vi "pullPatchByArc_v02.vi"(0 "manp in":T2={"Actuator COM"="COM6", "Actuator type"=enum."Scientifica"}, 1 "reset motion":T1=enum."slow_dualPatch", 5 "Current Position":i32[](array[numeric]), 7 "Steps":i32, 9 "Final Distance (steps)":i32, 11 "error in":errorcluster) -> (4 "manip out":T2={"Actuator COM"="COM14", "Actuator type"=enum."Scientifica"}, 15 "error out":errorcluster)   [LabVIEW 2019]
uses:
  pipette cleaning/pressure box/cleaning_soft/controls/actuator_cluster.ctl
  pipette cleaning/pressure box/cleaning_soft/controls/actuator_type.ctl
  controls/scope_motion.ctl
panel:
  out "positionSequence":i32[][](array[numeric])
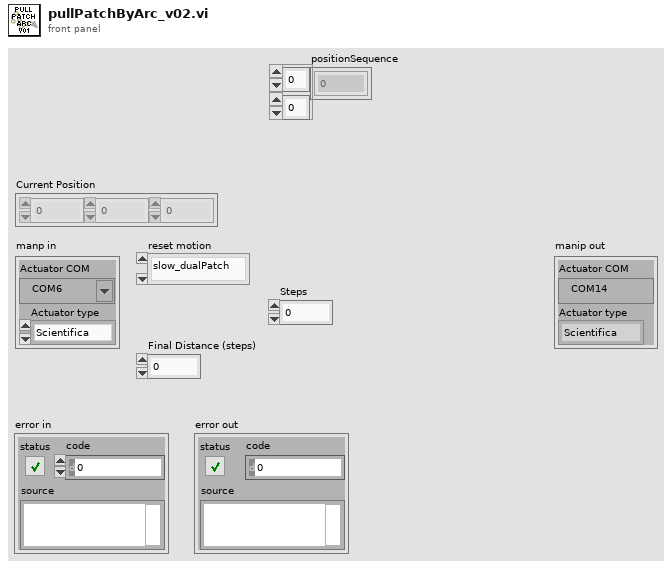
[diagram p1: front panel]
types:
  T1 = typedef "scope_motion.ctl" = enum16{"superSlow", "fast", "slow", "find slice speed", "slow_dualPatch"}
  T2 = typedef "actuator_cluster.ctl" = cluster{"Actuator COM":refnum<visa-resource-name>, "Actuator type":T3}
  T3 = typedef "actuator_type.ctl" = enum16{"Scientifica", "Sutter", "Demo", "Off"}
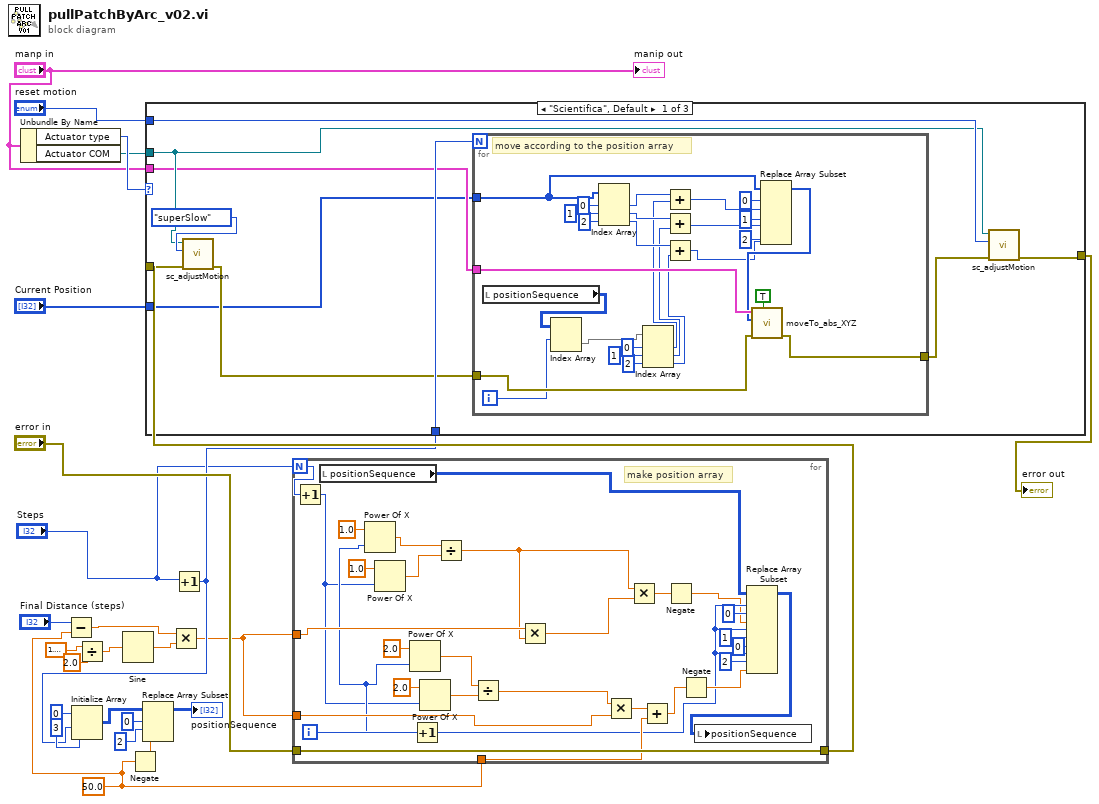
[diagram p0: block diagram]
diagram:
  w3 = 50.0 ("new element/subarray")
  n1 = Unbundle By Name("manp in") -> ("Actuator type"=w25:T3, "Actuator COM"=w24:refnum<visa-resource-name>)
  n2 = Subtract(x="Final Distance (steps)", y=w3) -> (x-y=w2:dbl)
  n3 = Divide(x=1.5707963267948966, y=2.0) -> (x/y=w12:dbl)
  n4 = Sine(x=w12) -> (sin(x)=w14:dbl)
  n5 = Negate(x=w3) -> (-x=w6:dbl)
  n6 = Multiply(x=w2, y=w14) -> (x*y=w8:dbl)
  n7 = Increment(x="Steps") -> (x+1=w9:i32)
  n8 = Initialize Array(0 ("element"), w9, 3 ("dimension size")) -> (w19:i32[][])
  n9 = Replace Array Subset(array=w19, new element=w6, index (row)=0 ("index"), index (col)=2 ("disabled index (col)")) -> (→"positionSequence":i32[][])
  n10 = for {
    N: "Steps" -> [w44]
    tunnel: w8 -> [w52]
    tunnel: "error in" -> [w50]
    tunnel: [w50] -> w10
    tunnel: w8 -> [w41]
    tunnel: w3 -> [w47]
    i -> [w43]
    # "make position array"
    n11 = Increment(x=w44) -> (x+1=w29:i32)
    n12 = local read "positionSequence"() -> (w49:i32[][])
    n13 = Power Of X(1:w29, 2:1.0 ("y")) -> (0:w34:dbl)
    n14 = Increment(x=w43) -> (x+1=w31:i32)
    n15 = Power Of X(1:w31, 2:1.0 ("y")) -> (0:w36:dbl)
    n16 = Power Of X(1:w31, 2:2.0 ("y")) -> (0:w30:dbl)
    n17 = Power Of X(1:w29, 2:2.0 ("y")) -> (0:w28:dbl)
    n18 = Divide(x=w36, y=w34) -> (x/y=w40:dbl)
    n19 = Divide(x=w30, y=w28) -> (x/y=w53:dbl)
    n20 = Multiply(x=w41, y=w40) -> (x*y=w39:dbl)
    n21 = Multiply(x=w53, y=w52) -> (x*y=w42:dbl)
    n22 = Multiply(x=w40, y=w39) -> (x*y=w48:dbl)
    n23 = Add(x=w42, y=w47) -> (x+y=w45:dbl)
    n24 = Negate(x=w48) -> (-x=w26:dbl)
    n25 = Negate(x=w45) -> (-x=w38:dbl)
    n26 = Replace Array Subset(array=w49, new element #1=w26, index (row) #1=w31, index (col) #1=0 ("index (row)"), new element #2=0 ("new element/subarray"), index (row) #2=w31, index (col) #2=1 ("disabled index (col)"), new element #3=w38, index (row) #3=w31, index (col) #3=2 ("disabled index (col)")) -> (w51:i32[][])
    n27 = local write "positionSequence"(w51) -> ()
  }
  n28 = case shown="\"Scientifica\", Default" w25 {
    tunnel: w24 -> [w61 _ _]
    tunnel: w10 -> [w65 w93 w94]
    tunnel: [w62 w93 w94] -> w22
    tunnel: "reset motion" -> [w64 _ _]
    tunnel: w9 -> [w60 _ _]
    tunnel: "Current Position" -> [w56 _ _]
    tunnel: "manp in" -> [w59 _ _]
    frame "Scientifica", Default {
      n29 = call "sc_adjustMotion.vi"("error in (no error)"=w65, "motion"=scope_motion."superSlow", "VISA handle"=w61) -> ("error out"=w58:errorcluster)  [unwired: 7 in, 1 out]
      n30 = for {
        N: w60 -> [_]
        tunnel: w59 -> [w92]
        tunnel: w58 -> [w90]
        tunnel: [w89] -> w57
        tunnel: w56 -> [w77]
        i -> [w79]
        # "move according to the position array"
        n31 = local read "positionSequence"() -> (w66:i32[][])
        n32 = Index Array(array=w66, index (row)=w79) -> (element=w73:i32[])  [unwired: 1 in]
        n33 = Index Array(array=w77, index #1=0 ("index"), index #2=1 ("index"), index #3=2 ("index")) -> (element #1=w82:i32, element #2=w81:i32, element #3=w80:i32)
        n34 = Index Array(array=w73, index #1=0 ("index"), index #2=1 ("index"), index #3=2 ("index")) -> (element #1=w70:i32, element #2=w72:i32, element #3=w71:i32)
        n35 = Add(x=w82, y=w70) -> (x+y=w67:i32)
        n36 = Add(x=w81, y=w72) -> (x+y=w68:i32)
        n37 = Add(x=w80, y=w71) -> (x+y=w69:i32)
        n38 = Replace Array Subset(array=w77, new element #1=w67, index #1=0 ("index"), new element #2=w68, index #2=1 ("index"), new element #3=w69, index #3=2 ("index")) -> (w78:i32[])
        n39 = call "moveTo_abs_XYZ.vi"("blocking?"=TRUE, "error in"=w90, "XYZ location (steps)"=w78, "Actuator cluster in"=w92) -> ("error out"=w89:errorcluster)  [unwired: 6 in, 1 out]
      }
      n40 = call "sc_adjustMotion.vi"("error in (no error)"=w57, "motion"=w64, "VISA handle"=w61) -> ("error out"=w62:errorcluster)  [unwired: 7 in, 1 out]
    }
    frame "Sutter" {
    }
    frame "Demo" {
    }
  }
  "error out" <- w22
  "manip out" <- "manp in"
